vi "get_ecrh_dur_from_json.vi"() -> ()   [LabVIEW 2014]
uses:
  <vilib>/regexp/Match Regular Expression.xnode
panel:
  out "number":dbl
  in  "body 2":string
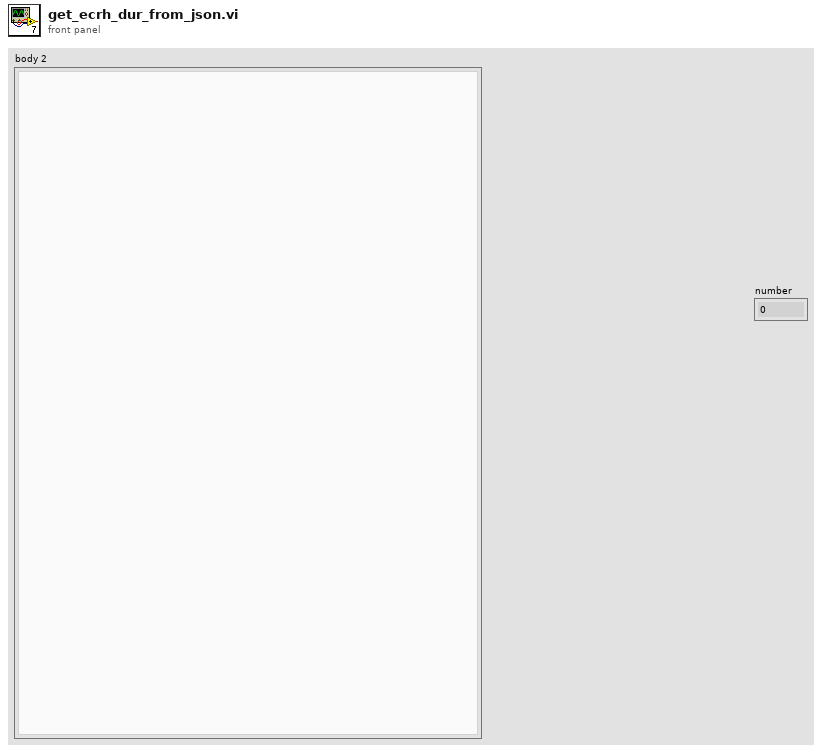
[diagram p1: front panel]
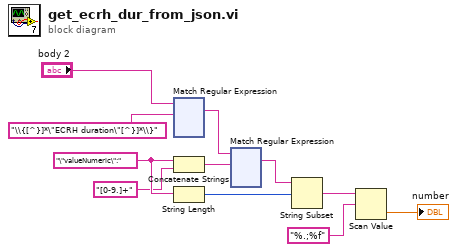
[diagram p0: block diagram]
diagram:
  w7 = "\"valueNumeric\":"
  n1 = xnode "Match Regular Expression"("input string"="body 2", "regular expression"="\\{[^}]*\"ECRH duration\"[^}]*\\}") -> ("whole match"=w9:string)  [unwired: 4 in, 4 out]
  n2 = Concatenate Strings(w7, "[0-9.]+") -> (w5:string)
  n3 = String Length(string=w7) -> (length=w8:i32)
  n4 = xnode "Match Regular Expression"("input string"=w9, "regular expression"=w5) -> ("whole match"=w4:string)  [unwired: 4 in, 4 out]
  n5 = String Subset(string=w4, offset (0)=w8) -> (substring=w3:string)  [unwired: 1 in]
  n6 = Scan Value(string=w3, format string="%.;%f") -> (value=→"number":dbl)  [unwired: 1 in, 1 out]
